vi "sc5511a_get_alc_dac.vi"(0 "deviceHandle":u32 format="%.0x", 5 "error in":errorcluster) -> (14 "deviceHandle":u32 format="%.0x", 16 "dac_value":u16, 19 "error out":errorcluster)   [LabVIEW 2010]
uses:
  sc5511a_rs232.dll
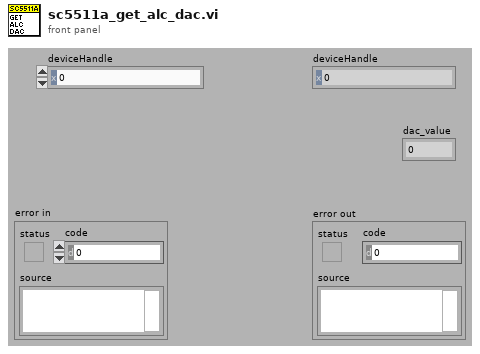
[diagram p1: front panel]
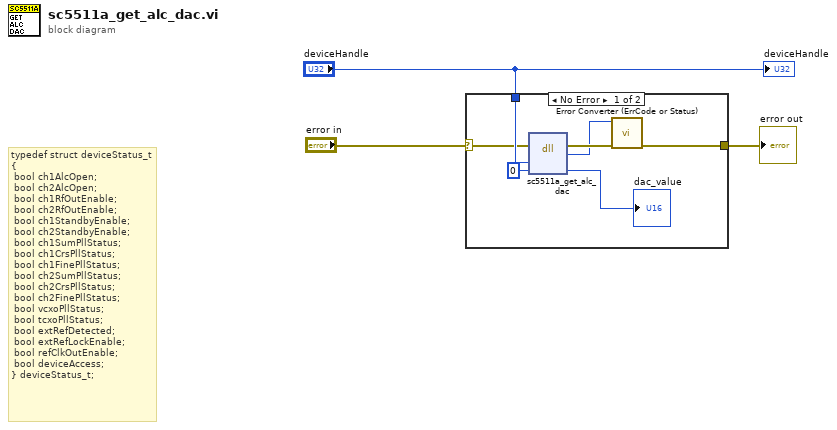
[diagram p0: block diagram]
diagram:
  # "typedef struct deviceStatus_t\n{\n\tbool ch1AlcOpen;\n\tbool ch2AlcOpen;\n\tbool ch1RfOutEnable;\n\tbool ch2RfOutEnable;\n\tbool ch1StandbyEnable;\t\t\t\t\t\n\tbool ch2StandbyEnable;\n\tbool ch1SumPllStatus;\n\tbool ch1CrsPllStatus;\n\tbool ch1FinePllStatus;\n\tbool ch2SumPllStatus;\n\tbool ch2CrsPllStatus;\n\tbool ch2FinePllStatus;\n\tbool vcxoPllStatus;\n\tbool tcxoPllStatus;\n\tbool extRefDetected;\n\tbool extRefLockEnable;\n\tbool refClkOutEnable;\n\tbool deviceAccess;\n}\tdeviceStatus_t;"
  n1 = case shown="No Error" "error in" {
    selector: "error in" -> [w4 w11]
    tunnel: [w10 w11] -> w2
    tunnel: "deviceHandle" -> [w7 _]
    frame No Error {
      n2 = dll-call lib="sc5511a_rs232.dll" fn="sc5511a_get_alc_dac"(error in=w4, "deviceHandle"=w7, "dac_value"=u16 0) -> (error out=w9:errorcluster, "return type"=w8:i32, "dac_value"=→"dac_value":u16)  [unwired: 3 in, 1 out]
      n3 = call "Error Converter (ErrCode or Status).vi"("error in (no error)"=w9, "error code"=w8) -> ("error out"=w10:errorcluster)  [unwired: 9 in]
    }
    frame Error {
    }
  }
  "error out" <- w2
  "deviceHandle" <- "deviceHandle"
